vi "leapSeconds LUT.vi"() -> (1 "Leap Seconds":i64[](array[numeric]), 3 "UTC Time":i64[](array[numeric]))   [LabVIEW 2018, in "Epoch.lvclass"]
uses:
  Epoch.lvclass
  <vilib>/regexp/Match Regular Expression.xnode
  <vilib>/Utility/miscctls.llb/LVDateTimeRec.ctl
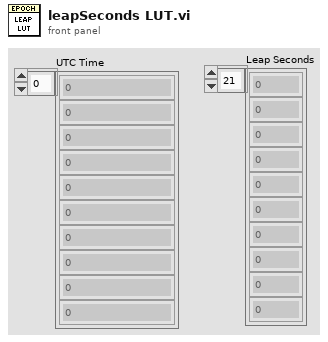
[diagram p1: front panel]
types:
  T1 = typedef "LVDateTimeRec.ctl" = cluster{"fractional second":dbl, "second":i32, "minute":i32, "hour":i32, "day of month":i32, "month":i32, "year":i32, "day of week":i32, "day of year":i32, "DST":i32}
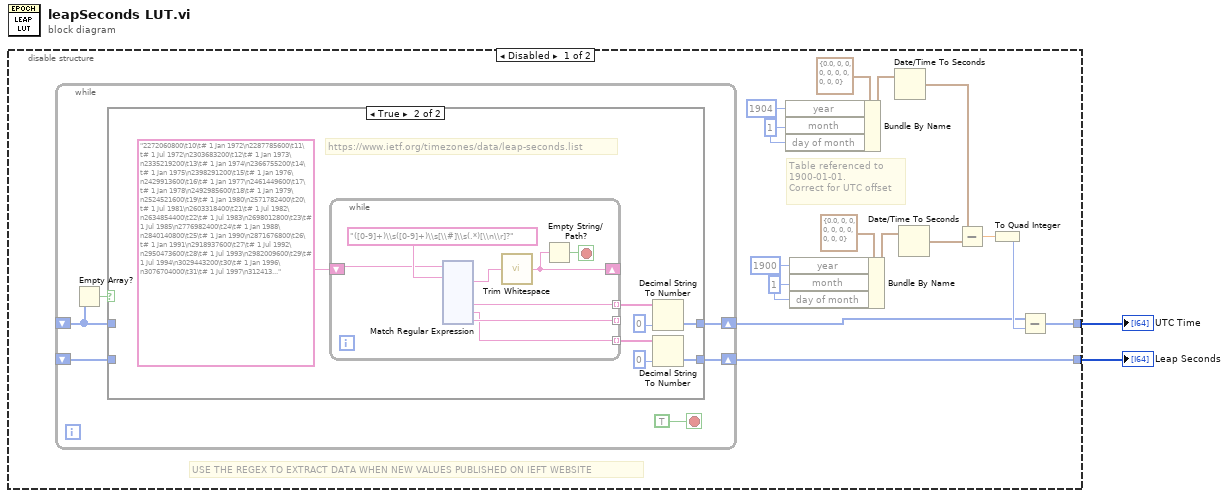
[diagram p0: block diagram]
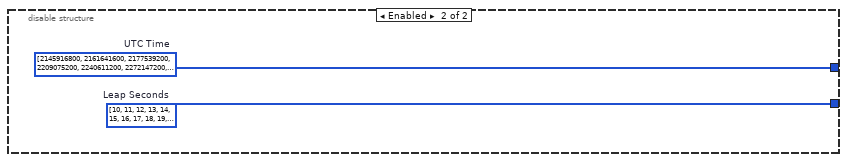
[diagram p3: hidden frame]
diagram:
  n1 = disable-structure shown="Disabled" {
    disable-tunnel: [w17 w160] -> w2
    disable-tunnel: [w13 w159] -> w1
    frame Disabled {
      w4 = 1 ("month")
      w12 = 1 ("month")
      # "Table referenced to \n1900-01-01.\nCorrect for UTC offset"
      # "USE THE REGEX TO EXTRACT DATA WHEN NEW VALUES PUBLISHED ON IEFT WEBSITE"
      n2 = while {
        shift-right: [w22] -> w14
        shift-left: _ -> [w19]
        shift-right: [w23] -> w17
        shift-left: _ -> [w18]
        stop <- TRUE stop-if-true
        n3 = Empty Array?(array=w19) -> (empty?=w20:bool)
        n4 = case shown="True" w20 {
          tunnel: [w24 w27] -> w23
          tunnel: [w25 w26] -> w22
          tunnel: w19 -> [w25 _]
          tunnel: w18 -> [w24 _]
          frame False {
          }
          frame True {
            # "https://www.ietf.org/timezones/data/leap-seconds.list"
            n5 = while {
              shift-right: [w38] -> _
              shift-left: "2272060800\t10\t# 1 Jan 1972\n2287785600\t11\t# 1 Jul 1972\n2303683200\t12\t# 1 Jan 1973\n2335219200\t13\t# 1 Jan 1974\n2366755200\t14\t# 1 Jan 1975\n2398291200\t15\t# 1 Jan 1976\n2429913600\t16\t# 1 Jan 1977\n2461449600\t17\t# 1 Jan 1978\n2492985600\t18\t# 1 Jan 1979\n2524521600\t19\t# 1 Jan 1980\n2571782400\t20\t# 1 Jul 1981\n2603318400\t21\t# 1 Jul 1982\n2634854400\t22\t# 1 Jul 1983\n2698012800\t23\t# 1 Jul 1985\n2776982400\t24\t# 1 Jan 1988\n2840140800\t25\t# 1 Jan 1990\n2871676800\t26\t# 1 Jan 1991\n2918937600\t27\t# 1 Jul 1992\n2950473600\t28\t# 1 Jul 1993\n2982009600\t29\t# 1 Jul 1994\n3029443200\t30\t# 1 Jan 1996\n3076704000\t31\t# 1 Jul 1997\n3124137600\t32\t# 1 Jan 1999\n3345062400\t33\t# 1 Jan 2006\n3439756800\t34\t# 1 Jan 2009\n3550089600\t35\t# 1 Jul 2012\n3644697600\t36\t# 1 Jul 2015\n3692217600\t37\t# 1 Jan 2017" -> [w36]
              tunnel: [w35] -> w31 mode=indexing
              tunnel: [w34] -> _ mode=indexing
              tunnel: [w33] -> w28 mode=indexing
              stop <- w39 stop-if-true
              n6 = xnode "Match Regular Expression"("input string"=w36, "regular expression"="([0-9]+)\\s([0-9]+)\\s[\\#]\\s(.*)[\\n\\r]?") -> ("after match"=w40:string, "submatch 1"=w35:string, "submatch 2"=w33:string, "submatch 3"=w34:string)  [unwired: 4 in, 4 out]
              n7 = call <vilib>:"Trim Whitespace.vi"("string"=w40) -> ("trimmed string"=w38:string)  [unwired: 1 in]
              n8 = Empty String/Path?(string/path=w38) -> (empty?=w39:bool)
            }
            n9 = Decimal String To Number(string=w31, default (0L)=i64 0 ("Epoch Time (s)")) -> (number=w26:i64[])  [unwired: 1 in, 1 out]
            n10 = Decimal String To Number(string=w28, default (0L)=i64 0 ("Epoch Time (s)")) -> (number=w27:i64[])  [unwired: 1 in, 1 out]
          }
        }
      }
      n11 = Bundle By Name(cluster=T1 {"fractional second"=0.0, "second"=0, "minute"=0, "hour"=0, "day of month"=0, "month"=0, "year"=0, "day of week"=0, "day of year"=0, "DST"=0} ("date time rec"), "year"=1904, "month"=w12, "day of month"=w12) -> (w10:T1)
      n12 = Bundle By Name(cluster=T1 {"fractional second"=0.0, "second"=0, "minute"=0, "hour"=0, "day of month"=0, "month"=0, "year"=0, "day of week"=0, "day of year"=0, "DST"=0} ("date time rec"), "year"=1900, "month"=w4, "day of month"=w4) -> (w6:T1)
      n13 = Date/Time To Seconds(2:w10) -> (0:w8:timestamp)  [unwired: 1 in]
      n14 = Date/Time To Seconds(2:w6) -> (0:w3:timestamp)  [unwired: 1 in]
      n15 = Subtract(x=w8, y=w3) -> (x-y=w16:dbl)
      n16 = To Quad Integer(1:w16) -> (0:w15:i64)
      n17 = Subtract(x=w14, y=w15) -> (x-y=w13:i64[])
    }
    frame Enabled {
      w160 = i64[] [10, 11, 12, 13, 14, 15, 16, 17, 18, 19, 20, 21, 22, 23, 24, 25, 26, 27, 28, 29, 30, 31, 32, 33, 34, 35, 36, 37]  # Leap Seconds
      w159 = i64[] [2145916800, 2161641600, 2177539200, 2209075200, 2240611200, 2272147200, 2303769600, 2335305600, 2366841600, 2398377600, 2445638400, 2477174400, 2508710400, 2571868800, 2650838400, 2713996800, 2745532800, 2792793600, 2824329600, 2855865600, 2903299200, 2950560000, 2997993600, 3218918400, 3313612800, 3423945600, 3518553600, 3566073600]  # UTC Time
    }
  }
  "Leap Seconds" <- w2
  "UTC Time" <- w1
